vi "Pre Launch Init.vi"(11 "DialogueM in":refnum<class "DialogueM.lvclass"> caption="操作者输入") -> (0 "error out":errorcluster caption="错误输出", 3 "DialogueM out":refnum<class "DialogueM.lvclass"> caption="操作者输出")   [LabVIEW 2014, in "DialogueManagement.lvlib" / "DialogueM.lvclass"]
doc: "(<B>Filename</B>: Actor Framework.lvlib:Actor.lvclass:Pre Launch Init.vi)\n\nDefines behavior that occurs after the Launch Nested Actor method is invoked but before the actor's Actor Core method begins running.\n\nBy default, this method does nothing. A descendant class may override it to define behavior."
uses:
  DialogueM.lvclass
  DialogueM.lvclass/DialogueM.ctl
  <vilib>/ActorFramework/Actor/Actor.lvclass
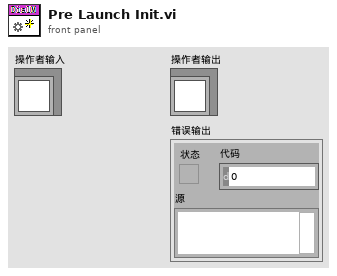
[diagram p1: front panel]
types:
  T1 = cluster{"Stop":refnum<user-event>, "Text":refnum<user-event>, "Connected":refnum<user-event>}
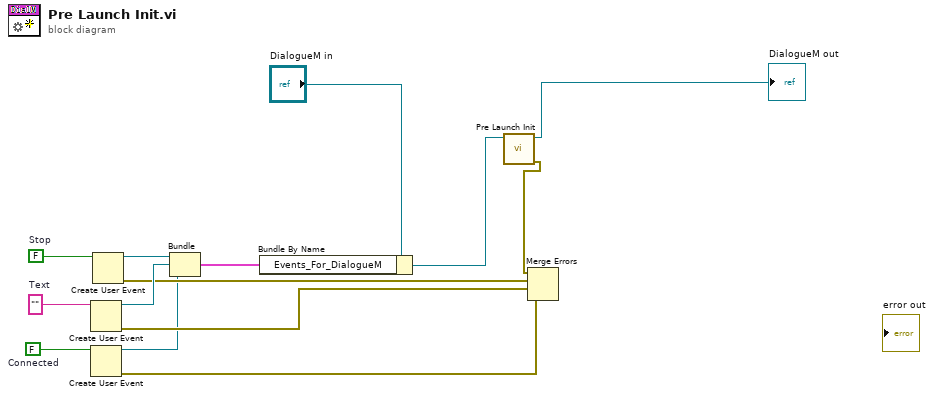
[diagram p0: block diagram]
diagram:
  w6 = FALSE  # Connected
  w12 = FALSE  # Stop
  w13 = ""  # Text
  n1 = Create User Event(user event datatype=w13) -> (user event=w10:refnum<user-event>, error out=w7:errorcluster)  [unwired: 1 in]
  n2 = Create User Event(user event datatype=w6) -> (user event=w4:refnum<user-event>, error out=w5:errorcluster)  [unwired: 1 in]
  n3 = Create User Event(user event datatype=w12) -> (user event=w11:refnum<user-event>, error out=w8:errorcluster)  [unwired: 1 in]
  n4 = Bundle("Stop"=w11, "Text"=w10, "Connected"=w4) -> (w9:T1)  [unwired: 1 in]
  n5 = Bundle By Name(cluster="DialogueM in", "Events_For_DialogueM"=w9) -> (w2:refnum<class "DialogueM.lvclass">)
  n6 = call-parent "Pre Launch Init.vi"("Actor in"=w2) -> ("error out"=w1:errorcluster, "Actor out"=→"DialogueM out":refnum<class "DialogueM.lvclass">)  [unwired: 9 in]
  n7 = Merge Errors(w1, w8, w7, w5) -> ()  [unwired: 1 out]
